vi "Esclavo_2.vi"() -> ()   [LabVIEW 2017]
uses:
  <vilib>/Modbus/slave/Create Slave Instance (TCP).vi
  <vilib>/Modbus/slave/Modbus Slave.lvclass
panel:
  in  "Sobrecarga Electrica":bool
  in  "Alarma de temperatura":bool
  in  "Modo Manual":bool
  in  "Boton de pánico":bool
  out "Variables de planta":u16[](array[numeric])
  in  "stop":bool
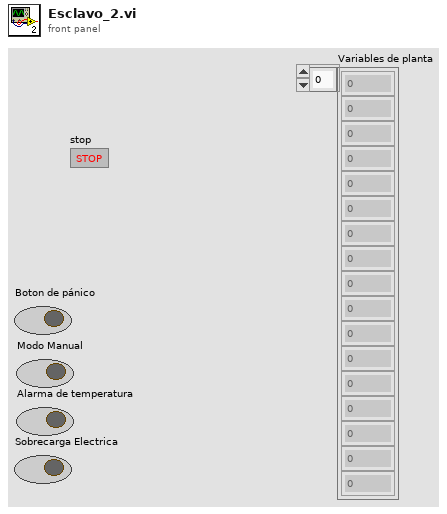
[diagram p1: front panel]
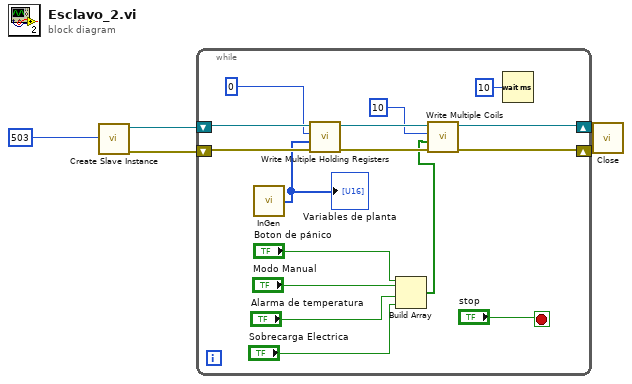
[diagram p0: block diagram]
diagram:
  n1 = call-poly <vilib>:"Create Slave Instance.vi"("port (502)"=u16 503) -> ("error out"=w4:errorcluster, "TCP slave instance"=w3:refnum<class "Modbus Slave.lvclass">)  [unwired: 9 in]
  n2 = while {
    shift-right: [w12] -> w1
    shift-left: w3 -> [w19]
    shift-right: [w13] -> w2
    shift-left: w4 -> [w18]
    stop <- "stop" stop-if-true
    n3 = call "InGen.vi"() -> ("Variables de planta"=w16:u16[])
    "Variables de planta" <- w16
    n4 = call-dynamic "Write Multiple Holding Registers.vi"("error in (no error)"=w18, "holding register values"=w16, "starting address"=u16 0, "Modbus slave in"=w19) -> ("error out"=w14:errorcluster, "Modbus slave out"=w15:refnum<class "Modbus Slave.lvclass">)  [unwired: 6 in]
    n5 = Build Array("Boton de pánico", "Modo Manual", "Alarma de temperatura", "Sobrecarga Electrica") -> (w6:bool[])
    n6 = call-dynamic "Write Multiple Coils.vi"("error in (no error)"=w14, "coil values"=w6, "starting address"=u16 10, "Modbus slave in"=w15) -> ("error out"=w13:errorcluster, "Modbus slave out"=w12:refnum<class "Modbus Slave.lvclass">)  [unwired: 6 in]
    n7 = Wait (ms)(milliseconds to wait=u32 10) -> ()  [unwired: 1 out]
  }
  n8 = call-dynamic "Close.vi"("error in (no error)"=w2, "Modbus slave in"=w1) -> ()  [unwired: 9 in, 1 out]
